vi "Delay if needed.vi"(6 "Modbus status":T1, 8 "error in":errorcluster, 9 "milliseconds to wait":u32=200, 11 "VISA resource name":refnum<visa-resource-name>) -> (0 "error out":errorcluster, 3 "VISA resource name out":refnum<visa-resource-name>)   [LabVIEW 2019]
uses:
  Request to talk.ctl
panel:
  out "waiting":dbl
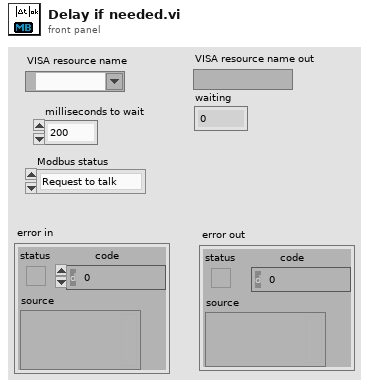
[diagram p1: front panel]
types:
  T1 = typedef "Request to talk.ctl" = enum16{"Request to talk", "Done"}
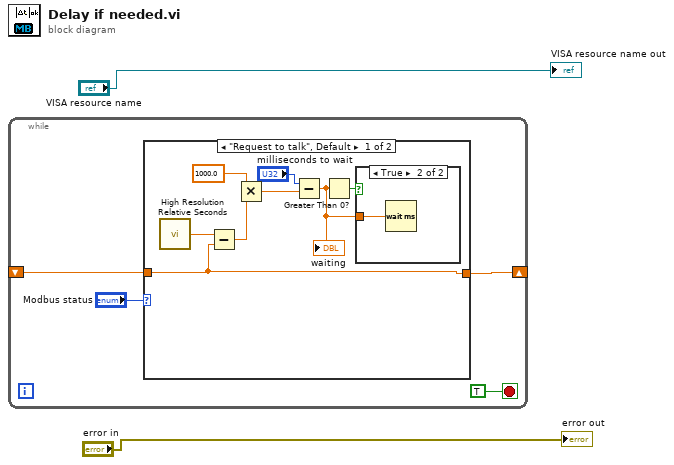
[diagram p0: block diagram]
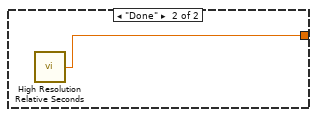
[diagram p3: hidden frame]
diagram:
  n1 = while {
    shift-right: [w4] -> _
    shift-left: _ -> [w3]
    stop <- TRUE stop-if-true
    n2 = case shown="\"Request to talk\", Default" "Modbus status" {
      tunnel: [w7 w16] -> w4
      tunnel: w3 -> [w7 _]
      frame "Request to talk", Default {
        n3 = call <vilib>:"High Resolution Relative Seconds.vi"() -> ("relative seconds"=w14:dbl)
        n4 = Subtract(x=w14, y=w7) -> (x-y=w13:dbl)
        n5 = Multiply(x=1000.0, y=w13) -> (x*y=w10:dbl)
        n6 = Subtract(x="milliseconds to wait", y=w10) -> (x-y=w8:dbl)
        "waiting" <- w8
        n7 = Greater Than 0?(x=w8) -> (x > 0?=w9:bool)
        n8 = case shown="True" w9 {
          tunnel: w8 -> [_ w15]
          frame False {
          }
          frame True {
            n9 = Wait (ms)(milliseconds to wait=w15) -> ()  [unwired: 1 out]
          }
        }
      }
      frame "Done" {
        n10 = call <vilib>:"High Resolution Relative Seconds.vi"() -> ("relative seconds"=w16:dbl)
      }
    }
  }
  "error out" <- "error in"
  "VISA resource name out" <- "VISA resource name"
